vi "function2.vi"(1 "y":dbl) -> (0 "x+y":dbl)   [LabVIEW 2012]
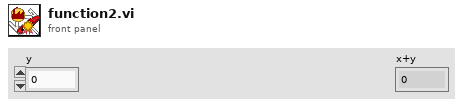
[diagram p1: front panel]
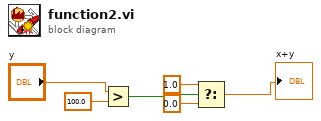
[diagram p0: block diagram]
diagram:
  n1 = Greater?(x="y", y=100.0) -> (0:w4:bool)
  n2 = Select(t=1.0, s=w4, f=0.0) -> (s? t:f=→"x+y":dbl)
